vi "HFRR ADV v07 new software.vi"() -> ()   [LabVIEW 2025] (continued)
            n281 = call <vilib>:"Clear Errors.vi"("error in (no error)"=w363) -> ()  [unwired: 5 in, 2 out]
          }
          frame True {
          }
        }
      }
      event "Heater Button": Value Change {
        n282 = event-data() -> ()  [unwired: 1 in, 6 out]
        n283 = local read "Heater Button"() -> (w381:bool)
        n284 = case shown="True" w381 {
          frame True {
            n285 = stacked-sequence {
              frame #0 {
                n286 = Wait (ms)(milliseconds to wait=u32 1500) -> ()  [unwired: 1 out]
              }
              frame #1 {
                n287 = local read "Set Temp"() -> (w383:dbl)
                n288 = Number To Fractional String(number=w383, precision (6)=i16 2) -> (F-format string=w386:string)  [unwired: 2 in]
                n289 = Concatenate Strings("ST;" ("Command"), w386) -> (w385:string)
                n290 = local write "Command"(w385) -> ()
              }
              frame #2 {
                n291 = Wait (ms)(milliseconds to wait=u32 1500) -> ()  [unwired: 1 out]
              }
              frame #3 {
                n292 = local write "Command"("HE;1" ("Command")) -> ()
              }
              frame #4 {
                n293 = Wait (ms)(milliseconds to wait=u32 1500) -> ()  [unwired: 1 out]
              }
            }
          }
          frame False {
            n294 = stacked-sequence {
              frame #0 {
                n295 = Wait (ms)(milliseconds to wait=u32 1500) -> ()  [unwired: 1 out]
              }
              frame #1 {
                n296 = Concatenate Strings("ST;" ("Command"), "0" ("string")) -> (w393:string)
                n297 = local write "Command"(w393) -> ()
              }
              frame #2 {
                n298 = Wait (ms)(milliseconds to wait=u32 1500) -> ()  [unwired: 1 out]
              }
              frame #3 {
                n299 = local write "Command"("HE;0" ("Command")) -> ()
              }
              frame #4 {
                n300 = Wait (ms)(milliseconds to wait=u32 1500) -> ()  [unwired: 1 out]
              }
            }
          }
        }
      }
      event "Headen Service Button": Value Change {
        n301 = event-data() -> ()  [unwired: 1 in, 6 out]
        n302 = local read "Headen Service Button"() -> (w398:bool)
        n303 = case shown="True" w398 {
          frame False {
            n304 = property on="Password 3" class="Clust (strict)"("Visible"=FALSE) -> ()  [unwired: 2 in, 2 out]
            n305 = property on="Service Password Log" class="Str"("Visible"=FALSE) -> ()  [unwired: 2 in, 2 out]
          }
          frame True {
            n306 = property on="Password 3" class="Clust (strict)"("Visible"=TRUE) -> ()  [unwired: 2 in, 2 out]
            n307 = property on="Service Password Log" class="Str"("Visible"=TRUE) -> ()  [unwired: 2 in, 2 out]
          }
        }
      }
      event "Password 3.Service Password": Value Change {
        n308 = event-data() -> ()  [unwired: 1 in, 6 out]
        n309 = Unbundle By Name("Password 3") -> ("Service Password"=w405:string)
        n310 = call <vilib>:"Trim Whitespace.vi"("string"=w405) -> ("trimmed string"=w403:string)  [unwired: 1 in]
        n311 = Equal?(x=w403, y="Service@123") -> (x = y?=w404:bool)
        n312 = case shown="False" w404 {
          selector: w404 -> [w409 w411]
          frame False {
            n313 = local write "Service Password enable"(w409) -> ()
            n314 = property on="Service Password Log" class="Str"("Visible"=TRUE) -> ()  [unwired: 2 in, 2 out]
            n315 = property on="Tab Control 5" class="TabCtl (strict)"("Tabs Visible?"=TRUE ("Page Labels Display Visible?")) -> ()  [unwired: 2 in, 2 out]
          }
          frame True {
            n316 = property on="Service Password Log" class="Str"("Visible"=FALSE) -> ()  [unwired: 2 in, 2 out]
            "Service Password enable" <- w411
          }
        }
      }
      event "Sign In": Value Change {
        w413 = FALSE ("Visible")
        n317 = event-data() -> ()  [unwired: 1 in, 6 out]
        n318 = property on="About" class="Clust (strict)"("Visible"=w413) -> ()  [unwired: 2 in, 2 out]
        n319 = property on="Password 3" class="Clust (strict)"("Visible"=w413) -> ()  [unwired: 2 in, 2 out]
        n320 = property on="Service Password Log" class="Str"("Visible"=FALSE) -> ()  [unwired: 2 in, 2 out]
      }
      event "Info": Value Change {
        n321 = event-data() -> ()  [unwired: 1 in, 6 out]
        n322 = local read "Info"() -> (w415:bool)
        n323 = case shown="False" w415 {
          frame False {
            n324 = property on="About" class="Clust (strict)"("Visible"=FALSE) -> ()  [unwired: 2 in, 2 out]
          }
          frame True {
            n325 = property on="About" class="Clust (strict)"("Visible"=TRUE) -> ()  [unwired: 2 in, 2 out]
          }
        }
      }
      event "Calibration": Value Change {
        n326 = event-data() -> ()  [unwired: 1 in, 6 out]
        n327 = local read "Calibration"() -> (w419:bool)
        n328 = case shown="False" w419 {
          frame False {
            n329 = property on="Calibration 2" class="TabCtl (strict)"("Visible"=FALSE) -> ()  [unwired: 2 in, 2 out]
            n330 = local write "Cal Password"("" ("Cal Password")) -> ()
          }
          frame True {
            n331 = property on="Calibration 2" class="TabCtl (strict)"("Visible"=TRUE) -> ()  [unwired: 2 in, 2 out]
            n332 = local write "Cal Password"("" ("Cal Password")) -> ()
          }
        }
        n333 = property on="Wrong Password" class="Str"("Visible"=FALSE) -> ()  [unwired: 2 in, 2 out]
      }
      event "Cal Password": Value Change {
        n334 = event-data() -> ()  [unwired: 1 in, 6 out]
        n335 = local read "Cal Password"() -> (w427:string)
        n336 = call <vilib>:"Trim Whitespace.vi"("string"=w427) -> ("trimmed string"=w426:string)  [unwired: 1 in]
        n337 = Equal?(x=w426, y="Cal@321") -> (x = y?=w424:bool)
        n338 = case shown="True" w424 {
          frame False {
            n339 = property on="Wrong Password" class="Str"("Visible"=TRUE) -> ()  [unwired: 2 in, 2 out]
          }
          frame True {
            n340 = property on="Wrong Password" class="Str"("Visible"=FALSE) -> ()  [unwired: 2 in, 2 out]
            n341 = local write "Main Tab"(T2."About" ("Main Tab")) -> ()
            n342 = local write "Cal Password"("" ("Cal Password")) -> ()
            n343 = local write "Main Dashboard Buttons"(T1."About" ("Main Dashboard Buttons")) -> ()
            n344 = local write "Tab Control 5"(T9."Temperature Calibration" ("Tab Control 5")) -> ()
            n345 = property on="Calibration 2" class="TabCtl (strict)"("Visible"=FALSE) -> ()  [unwired: 2 in, 2 out]
            n346 = property on="Tab Control 5" class="TabCtl (strict)"("Tabs Visible?"=FALSE ("Page Labels Display Visible?")) -> ()  [unwired: 2 in, 2 out]
            n347 = local write "Calibration"(FALSE ("Calibration")) -> ()
          }
        }
      }
      event "Quit": Value Change {
        n348 = event-data() -> ()  [unwired: 1 in, 6 out]
      }
    }
    n349 = Wait (ms)(milliseconds to wait=u32 100) -> ()  [unwired: 1 out]
  }
  n350 = local write "Auto stop temp"(w14) -> ()
  n351 = local write "main tab sub"(enum32{"Page 1", "Page 2"}."Page 1" ("main tab sub")) -> ()
  n352 = local write "USERNAME"(w31) -> ()
  n353 = local write "Main Tab"(T2."HOME" ("Main Tab")) -> ()
  n354 = local write "USER ID"(w31) -> ()
  n355 = property on="Auto Scar Check  2" class="Clust (strict)"("Visible"=w14) -> (error out=w17:errorcluster)  [unwired: 2 in, 1 out]
  n356 = property on="Quit" class="Bool (strict)"("Value"=FALSE ("Quit")) -> (error out=w33:errorcluster)  [unwired: 2 in, 1 out]
  n357 = while {
    shift-right: [w439] -> _
    shift-left: "Enum - Selector" -> [w440]
    stop <- w441 stop-if-true
    # "Auto Start Logic Loop"
    n358 = case shown="\"close\"" w440 {
      tunnel: [w444 w450 w462 w494 w525 Auto_Start_enum."Exit" ("Enum - Selector") Auto_Start_enum."Init" ("Enum - Selector")] -> w439
      frame "Init", Default {
        n359 = local read "Auto Start Test"() -> (w443:bool)
        n360 = Select(t=Auto_Start_enum."Humidity & Temperature On" ("Enum - Selector"), s=w443, f=Auto_Start_enum."Init") -> (s? t:f=w444:T12)
      }
      frame "Humidity & Temperature On" {
        n361 = flat-sequence {
          tunnel: [Auto_Start_enum."Reach point" ("Enum - Selector")] -> w447
          frame #0 {
            w452 = T15."Disabled and Grayed Out" ("Disabled")
            w453 = TRUE ("Heater Button")
            n362 = property on="Humidity" class="Bool (strict)"("DisabledEnum"=w452) -> ()  [unwired: 2 in, 2 out]
            n363 = property on="Heater Button" class="Bool (strict)"("DisabledEnum"=w452) -> ()  [unwired: 2 in, 2 out]
            n364 = local write "Heater Button"(w453) -> ()
            n365 = local write "Humidity"(w453) -> ()
            n366 = property on="Heater Button" class="Bool (strict)"("Val(Sgnl)"=TRUE ("Value (Signaling)")) -> ()  [unwired: 2 in, 2 out]
          }
          frame #1 {
            n367 = Wait (ms)(milliseconds to wait=u32 3000) -> ()  [unwired: 1 out]
          }
          frame #2 {
            w455 = TRUE ("Reach point temp")
            n368 = local write "Reach point Humidity"(w455) -> ()
            n369 = local write "Reach point temp"(w455) -> ()
          }
        }
        n370 = local read "Auto Start Test"() -> (w449:bool)
        n371 = Not(x=w449) -> (.not. x?=w448:bool)
        n372 = Select(t=Auto_Start_enum."close", s=w448, f=w447) -> (s? t:f=w450:T12)
      }
      frame "Reach point" {
        w463 = TRUE ("PAUSE")
        w471 = 1.0 ("y")
        w474 = 1.0 ("y")
        n373 = local read "Set Temperature:"() -> (w475:dbl)
        n374 = local read "Set Humidity:"() -> (w470:dbl)
        n375 = local read "Humidity ( %RH )"() -> (w476:dbl)
        n376 = Add(x=w475, y=w474) -> (x+y=w473:dbl)
        n377 = Subtract(x=w475, y=w474) -> (x-y=w472:dbl)
        n378 = Add(x=w470, y=w471) -> (x+y=w469:dbl)
        n379 = Subtract(x=w470, y=w471) -> (x-y=w468:dbl)
        n380 = local read "TEMP"() -> (w477:dbl)
        n381 = In Range and Coerce(upper limit=w469, x=w476, lower limit=w468) -> (In Range?=w457:bool)  [unwired: 1 out]
        n382 = In Range and Coerce(upper limit=w473, x=w477, lower limit=w472) -> (In Range?=w458:bool)  [unwired: 1 out]
        n383 = case shown="True" w457 {
          frame False {
          }
          frame True {
            n384 = case shown="True" "Reach point Humidity" {
              selector: "Reach point Humidity" -> [_ w483]
              frame False {
              }
              frame True {
                n385 = local read "EVENT LOG"() -> (w480:string)
                n386 = Not(x=w483) -> (.not. x?=w482:bool)
                n387 = local write "Reach point Humidity"(w482) -> ()
                n388 = call "Event Log.vi"("Content"="Target Humidity reached", "EVENT LOG"=w480) -> ("EVENT LOG"=w481:string)  [unwired: 8 in, 1 out]
                n389 = local write "EVENT LOG"(w481) -> ()
              }
            }
          }
        }
        n390 = case shown="True" w458 {
          frame False {
          }
          frame True {
            n391 = case shown="True" "Reach point temp" {
              selector: "Reach point temp" -> [_ w489]
              frame False {
              }
              frame True {
                n392 = local read "EVENT LOG"() -> (w486:string)
                n393 = Not(x=w489) -> (.not. x?=w488:bool)
                n394 = local write "Reach point temp"(w488) -> ()
                n395 = call "Event Log.vi"("Content"="Target Temperature reached", "EVENT LOG"=w486) -> ("EVENT LOG"=w487:string)  [unwired: 8 in, 1 out]
                n396 = local write "EVENT LOG"(w487) -> ()
              }
            }
          }
        }
        n397 = local read "Auto Start Test"() -> (w461:bool)
        n398 = And(x=w458, y=w457) -> (x .and. y?=w467:bool)
        n399 = Select(t=Auto_Start_enum."Maintain Stage" ("Enum - Selector"), s=w467, f=Auto_Start_enum."Reach point" ("Enum - Selector")) -> (s? t:f=w464:T12)
        n400 = Not(x=w461) -> (.not. x?=w460:bool)
        n401 = Select(t=Auto_Start_enum."close", s=w460, f=w464) -> (s? t:f=w462:T12)
        n402 = call "ELAPSED TIMER VI.vi"("RESET"=w463, "PAUSE"=w463) -> ()  [unwired: 7 in, 3 out]
      }
      frame "Maintain Stage" {
        w503 = 2.0 ("y")
        w502 = 1.0 ("y")
        # "Humidity and  temperatures Set Point  have been reached"
        n403 = local read "Set Temperature:"() -> (w509:dbl)
        n404 = local read "Set Humidity:"() -> (w506:dbl)
        n405 = local read "Humidity ( %RH )"() -> (w510:dbl)
        n406 = Add(x=w509, y=w502) -> (x+y=w508:dbl)
        n407 = Subtract(x=w509, y=w502) -> (x-y=w507:dbl)
        n408 = local read "TEMP"() -> (w511:dbl)
        n409 = Add(x=w506, y=w503) -> (x+y=w505:dbl)
        n410 = Subtract(x=w506, y=w503) -> (x-y=w504:dbl)
        n411 = In Range and Coerce(upper limit=w508, x=w511, lower limit=w507) -> (In Range?=w501:bool)  [unwired: 1 out]
        n412 = In Range and Coerce(upper limit=w505, x=w510, lower limit=w504) -> (In Range?=w500:bool)  [unwired: 1 out]
        n413 = And(x=w501, y=w500) -> (x .and. y?=w499:bool)
        n414 = Not(x=w499) -> (.not. x?=w498:bool)
        n415 = call "ELAPSED TIMER VI.vi"("TARGET"=60.0, "RESET"=w498, "PAUSE"=FALSE) -> ("ELAPSED INDICATION"=w495:bool)  [unwired: 6 in, 2 out]
        n416 = case shown="True" w495 {
          tunnel: w495 -> [_ w514]
          tunnel: [Auto_Start_enum."Maintain Stage" ("Enum - Selector") w513] -> w493
          frame False {
          }
          frame True {
            n417 = stacked-sequence {
              tunnel: w514 -> [_ _ _ _ _]
              tunnel: [_ _ _ _ Auto_Start_enum."Start Stage" ("Enum - Selector")] -> w513
              frame #0 {
                n418 = local read "EVENT LOG"() -> (w516:string)
                n419 = call "Event Log.vi"("Content"="Humidity and temperature set point has stabilized.", "EVENT LOG"=w516) -> ("EVENT LOG"=w517:string)  [unwired: 8 in, 1 out]
                n420 = local write "EVENT LOG"(w517) -> ()
              }
              frame #1 {
                n421 = Wait (ms)(milliseconds to wait=u32 100) -> ()  [unwired: 1 out]
              }
              frame #2 {
                n422 = local read "EVENT LOG"() -> (w520:string)
                n423 = call "Event Log.vi"("Content"="Auto Test Started", "EVENT LOG"=w520) -> ("EVENT LOG"=w521:string)  [unwired: 8 in, 1 out]
                n424 = local write "EVENT LOG"(w521) -> ()
              }
              frame #3 {
                w522 = TRUE ("RUN")
                n425 = local write "RUN"(w522) -> ()
                "Auto Start Temp" <- w522
              }
              frame #4 {
              }
            }
          }
        }
        n426 = local read "Auto Start Test"() -> (w492:bool)
        n427 = Not(x=w492) -> (.not. x?=w491:bool)
        n428 = Select(t=Auto_Start_enum."close", s=w491, f=w493) -> (s? t:f=w494:T12)
      }
      frame "Start Stage" {
        w524 = TRUE ("PAUSE")
        n429 = local read "Auto Start Test"() -> (w529:bool)
        n430 = Not(x=w529) -> (.not. x?=w528:bool)
        n431 = Select(t=Auto_Start_enum."close" ("Enum - Selector"), s=w528, f=Auto_Start_enum."Start Stage" ("Enum - Selector")) -> (s? t:f=w525:T12)
        n432 = call "ELAPSED TIMER VI.vi"("RESET"=w524, "PAUSE"=w524) -> ()  [unwired: 7 in, 3 out]
      }
      frame "close" {
        w531 = FALSE ("Heater Button")
        n433 = local write "RUN"(w531) -> ()
        n434 = local write "Heater Button"(w531) -> ()
        n435 = local write "Humidity"(w531) -> ()
        n436 = local write "Auto Start Test"(w531) -> ()
        n437 = property on="Heater Button" class="Bool (strict)"("Val(Sgnl)"=FALSE ("Value (Signaling)")) -> ()  [unwired: 2 in, 2 out]
      }
      frame "Exit" {
      }
    }
    n438 = Wait (ms)(milliseconds to wait=u32 100) -> ()  [unwired: 1 out]
    n439 = local read "Quit"() -> (w441:bool)
  }
  n440 = property on="Service Password Log" class="Str"("Visible"=w14) -> ()  [unwired: 2 in, 2 out]
  n441 = property on="Password 3" class="Clust (strict)"("Visible"=w14) -> ()  [unwired: 2 in, 2 out]
  n442 = while {
    stop <- w560 stop-if-true
    w543 = errorcluster {"status"=FALSE, "code"=0, "source"=""} ("error in (no error) 3")
    # "this loop is for manual report generation"
    n443 = local read "Confirm Measrurement"() -> (w542:bool)
    n444 = case shown="True" w542 {
      selector: w542 -> [_ w650]
      tunnel: errorcluster {"status"=FALSE, "code"=0, "source"=""} ("error in (no error) 3") -> [_ w651]
      tunnel: [_ w649] -> _
      frame False {
      }
      frame True {
        n445 = stacked-sequence {
          tunnel: w651 -> [_ w684 _]
          tunnel: w650 -> [_ _ w791]
          tunnel: [_ w672 _] -> w649
          frame #0 {
            n446 = String To Path(string="C:\\LAB-IQ\\Image Calibrate v01.dcf") -> (path=w654:path)
            n447 = Open/Create/Replace File ("Open File")(file path (use dialog)=w654) -> (refnum out=w655:refnum<file>)  [unwired: 5 in, 2 out]
            n448 = for {
              N: 4 -> [_]
              tunnel: w655 -> [w661]
              i -> [w657]
              n449 = Read from Text File ("Read File")(file (use dialog)=w661) -> (text=w662:string)  [unwired: 3 in, 3 out]
              n450 = String Subset(string=w662, offset (0)=6, length (rest)=10 ("length (rest)")) -> (substring=w658:string)
              n451 = Fract/Exp String To Number(string=w658) -> (number=w656:dbl)  [unwired: 3 in, 1 out]
              n452 = case shown="3" w657 {
                tunnel: w656 -> [w663 w664 _ w665 _]
                frame 0 {
                  n453 = local write "5x Gain"(w663) -> ()
                }
                frame 1 {
                  n454 = local write "10x Gain"(w664) -> ()
                }
                frame 2 {
                }
                frame 3 {
                  n455 = local write "100x gain"(w665) -> ()
                }
                frame 4, Default {
                }
              }
            }
          }
          frame #1 {
            n456 = local read "TEST STANDARD"() -> (w667:T3)
            n457 = case shown="\"ISO 12156\"" w667 {
              tunnel: ["ASTM D6079" "ISO 12156"] -> w666
              frame "ASTM D6079", Default {
              }
              frame "ISO 12156" {
              }
            }
            n458 = call "IMAGE ANALYSIS.vi"("Enum"=POST_ANALYSIS_ENUM."GET MEASUREMENTS", "error in"=w684) -> ("error out"=w691:errorcluster)  [unwired: 8 in, 1 out]
            n459 = local read "Magnification :"() -> (w677:string)
            n460 = call "Stall Data Flow.vim"("value in"=w691, "milliseconds to wait"=u32 1000) -> ("value out"=w690:errorcluster)  [unwired: 1 out]
            n461 = local read "Test File List :"() -> (w688:string)
            n462 = case shown="\"10x\"" w677 {
              tunnel: [w727 w728] -> w675
              frame "5x", Default {
                n463 = local read "5x Gain"() -> (w727:dbl)
              }
              frame "10x" {
                # "5x"
                n464 = local read "10x Gain"() -> (w728:dbl)
              }
            }
            n465 = call "IMAGE ANALYSIS.vi"("Enum"=POST_ANALYSIS_ENUM."READ", "error in"=w690) -> ("error out"=w687:errorcluster, "data out"=w678:string)  [unwired: 8 in]
            n466 = Match Pattern(string=w678, regular expression="\"type\": ") -> (after substring=w682:string)  [unwired: 1 in, 3 out]
            n467 = call "IMAGE PATH CREATION PY.vi"("error in (no error)"=w687, "File Name :"=w688) -> ("error out"=w686:errorcluster, "File Path"=w674:path, "File Path String:"=w669:string)  [unwired: 7 in]
            n468 = Match Pattern(string=w682, regular expression=",") -> (before substring=w668:string)  [unwired: 1 in, 3 out]
            n469 = local read "Calibration Tab"() -> (w671:enum32{"Measrument", "Calibrate"})
            n470 = call "Stall Data Flow.vim"("value in"=w686, "milliseconds to wait"=u32 250) -> ("value out"=w670:errorcluster)  [unwired: 1 out]
            n471 = Equal?(x=w668, y="\"rectangle\"") -> (x = y?=w679:bool)
            n472 = case shown="False" w679 {
              tunnel: w678 -> [w733 w788]
              tunnel: w675 -> [_ w779]
              tunnel: cluster{"major":dbl, "minor":dbl, "average":dbl} {"major"=0.0, "minor"=0.0, "average"=0.0} -> [w731 w775]
              tunnel: [w730 w772] -> w673
              tunnel: w668 -> [w732 _]
              tunnel: w675 -> [w729 _]
              frame False {
                n473 = Equal?(x=w732, y="\"line\"") -> (x = y?=w734:bool)
                n474 = case shown="True" w734 {
                  tunnel: w733 -> [_ w749]
                  tunnel: w731 -> [w736 w748]
                  tunnel: [w736 w746] -> w730
                  tunnel: w729 -> [_ w745]
                  frame False {
                  }
                  frame True {
                    w744 = 0.0 ("Major Axis")
                    n475 = Match Pattern(string=w749, regular expression="\"length_px\":") -> (after substring=w747:string)  [unwired: 1 in, 3 out]
                    n476 = property on="Major Axis" class="DigNum (strict)"("Caption.Text"="") -> ()  [unwired: 2 in, 2 out]
                    n477 = property on="Minor Axis" class="DigNum (strict)"("Caption.Text"="") -> ()  [unwired: 2 in, 2 out]
                    n478 = property on="Average" class="DigNum (strict)"("Caption.Text"="Line") -> ()  [unwired: 2 in, 2 out]
                    n479 = Fract/Exp String To Number(string=w747, default (0 dbl)=0.0 ("default (0 DBL)")) -> (number=w743:dbl)  [unwired: 2 in, 1 out]
                    "Pixel Value" <- w743
                    n480 = Multiply(x=w743, y=w745) -> (x*y=w756:dbl)
                    n481 = Multiply(x=w756, y=1000.0) -> (x*y=w739:dbl)
                    n482 = Divide(x=w739, y=1000.0) -> (x/y=w742:dbl)
                    n483 = local write "Measurment (mm)"(w742) -> ()
                    n484 = Bundle By Name(cluster=w748, "average"=w739) -> (w746:cluster{"major":dbl, "minor":dbl, "average":dbl})
                    n485 = Number To Fractional String(number=w739, precision (6)=i16 1) -> (F-format string=w738:string)  [unwired: 2 in]
                    n486 = local write "Minor Axis"(w744) -> ()
                    n487 = local write "Major Axis"(w744) -> ()
                    n488 = Fract/Exp String To Number(string=w738) -> (number=w737:dbl)  [unwired: 3 in, 1 out]
                    n489 = local write "Average"(w737) -> ()
                  }
                }
              }
              frame True {
                w776 = 1000.0 ("y")
                w782 = 0.0 ("default (0 DBL)")
                n490 = Match Pattern(string=w788, regular expression=" \"width_px\":") -> (after substring=w786:string)  [unwired: 1 in, 3 out]
                n491 = Match Pattern(string=w786, regular expression="\"height_px\":") -> (before substring=w784:string, after substring=w783:string)  [unwired: 1 in, 2 out]
                n492 = Fract/Exp String To Number(string=w784, default (0 dbl)=w782) -> (number=w781:dbl)  [unwired: 2 in, 1 out]
                n493 = Fract/Exp String To Number(string=w783, default (0 dbl)=w782) -> (number=w780:dbl)  [unwired: 2 in, 1 out]
                n494 = Multiply(x=w781, y=w779) -> (x*y=w778:dbl)
                n495 = Multiply(x=w780, y=w779) -> (x*y=w777:dbl)
                n496 = Multiply(x=w778, y=w776) -> (x*y=w762:dbl)
                n497 = Multiply(x=w777, y=w776) -> (x*y=w760:dbl)
                n498 = Add(x=w762, y=w760) -> (x+y=w774:dbl)
                n499 = property on="Major Axis" class="DigNum (strict)"("Caption.Text"="Major Axis") -> ()  [unwired: 2 in, 2 out]
                n500 = property on="Minor Axis" class="DigNum (strict)"("Caption.Text"="Minor Axis") -> ()  [unwired: 2 in, 2 out]
                n501 = property on="Average" class="DigNum (strict)"("Caption.Text"="Average") -> ()  [unwired: 2 in, 2 out]
                n502 = Divide(x=w774, y=2.0) -> (x/y=w758:dbl)
                n503 = Bundle By Name(cluster=w775, "major"=w762, "minor"=w760, "average"=w758) -> (w772:cluster{"major":dbl, "minor":dbl, "average":dbl})
                n504 = Number To Fractional String(number=w760, precision (6)=i16 1) -> (F-format string=w767:string)  [unwired: 2 in]
                n505 = Number To Fractional String(number=w758, precision (6)=i16 1) -> (F-format string=w768:string)  [unwired: 2 in]
                n506 = Number To Fractional String(number=w762, precision (6)=i16 1) -> (F-format string=w766:string)  [unwired: 2 in]
                n507 = Fract/Exp String To Number(string=w767) -> (number=w759:dbl)  [unwired: 3 in, 1 out]
                n508 = Fract/Exp String To Number(string=w768) -> (number=w757:dbl)  [unwired: 3 in, 1 out]
                n509 = Fract/Exp String To Number(string=w766) -> (number=w761:dbl)  [unwired: 3 in, 1 out]
                n510 = local write "Major Axis"(w761) -> ()
                n511 = local write "Average"(w757) -> ()
                n512 = local write "Minor Axis"(w759) -> ()
              }
            }
            n513 = case shown="\"Measrument\", Default" w671 {
              tunnel: w674 -> [w701 _]
              tunnel: w673 -> [w700 _]
              tunnel: [w697 w726] -> w672
              tunnel: w670 -> [w699 w726]
              tunnel: w669 -> [w698 _]
              tunnel: w666 -> [w696 _]
              frame "Measrument", Default {
                n514 = stacked-sequence {
                  tunnel: w701 -> [w719 _]
                  tunnel: w700 -> [w717 _]
                  tunnel: w699 -> [w715 _]
                  tunnel: w698 -> [w714 _]
                  tunnel: [w709 _] -> w697
                  tunnel: w696 -> [w702 _]
                  frame #0 {
                    n515 = call "IMAGE ANALYSIS.vi"("Enum"=POST_ANALYSIS_ENUM."SAVE IMAGE", "error in"=w715, "IMAGE FILE PATH"=w714) -> ("error out"=w713:errorcluster)  [unwired: 7 in, 1 out]
                    n516 = call "Stall Data Flow.vim"("value in"=w713, "milliseconds to wait"=u32 1000) -> ("value out"=w704:errorcluster)  [unwired: 1 out]
                    n517 = local read "Test File List :"() -> (w721:string)
                    n518 = call "IMAGE ANALYSIS.vi"("Enum"=POST_ANALYSIS_ENUM."MINIMIZE UI", "error in"=w704) -> ("error out"=w711:errorcluster)  [unwired: 8 in, 1 out]
                    n519 = Bundle By Name(cluster=T22 {"File Name"="", "Test Method"="", "Operator"="", "Fuel Description"="", "Date and time"=""} ("Main Ref"), "Test Method"=w702, "File Name"=w721) -> (w722:T22)
                    n520 = call "Stall Data Flow.vim"("value in"=w711, "milliseconds to wait"=u32 1500) -> ("value out"=w706:errorcluster)  [unwired: 1 out]
                    n521 = call "duf file read.vi"("error in (no error)"=w706, "Main Ref"=w722) -> ("error out"=w720:errorcluster, "Main Ref 2"=w718:T22)  [unwired: 8 in]
                    n522 = call "DETECTION REPORT for manual.vi"("error in (no error)"=w720, "return value 3"=w717, "Image File Path"=w719, "Main Ref"=w718) -> ("error out"=w716:errorcluster)  [unwired: 7 in]
                    n523 = call <vilib>:"Clear Errors.vi"("error in (no error)"=w716) -> ("error out"=w707:errorcluster)  [unwired: 5 in, 1 out]
                    n524 = call "IMAGE ANALYSIS.vi"("Enum"=POST_ANALYSIS_ENUM."MINIMIZE UI", "error in"=w707) -> ("error out"=w709:errorcluster)  [unwired: 8 in, 1 out]
                  }
                  frame #1 {
                    n525 = local write "Main Tab"(T2."HOME" ("Main Tab")) -> ()
                    n526 = local write "Main Dashboard Buttons"(T1."Home" ("Main Dashboard Buttons")) -> ()
                  }
                }
              }
              frame "Calibrate" {
              }
            }
          }
          frame #2 {
            n527 = Not(x=w791) -> (.not. x?=w790:bool)
            n528 = local write "Confirm Measrurement"(w790) -> ()
            n529 = local read "Calibration Tab"() -> (w789:enum32{"Measrument", "Calibrate"})
            n530 = case shown="\"Measrument\", Default" w789 {
              frame "Measrument", Default {
                (unwired) T17."HOME" ("Main Tab")
                n531 = local write "Main Tab"(T2."HOME" ("Main Tab")) -> ()
              }
              frame "Calibrate" {
              }
            }
          }
        }
      }
    }
    n532 = local read "Humidity"() -> (w534:bool)
    n533 = local read "Save Change"() -> (w539:bool)
    n534 = local read "Calibrate"() -> (w540:bool)
    n535 = local read "Auto Start Test"() -> (w535:bool)
    n536 = case shown="True" w540 {
      selector: w540 -> [_ w647]
      frame False {
      }
      frame True {
        n537 = Not(x=w647) -> (.not. x?=w646:bool)
        n538 = local write "Calibrate"(w646) -> ()
        n539 = local write "Calibration Tab"(enum32{"Measrument", "Calibrate"}."Calibrate" ("Calibration Tab")) -> ()
      }
    }
    n540 = case shown="True" w539 {
      selector: w539 -> [_ w591]
      frame False {
      }
      frame True {
        n541 = stacked-sequence {
          tunnel: w591 -> [_ _ _ _ w645]
          frame #0 {
            n542 = call "IMAGE ANALYSIS.vi"("Enum"=POST_ANALYSIS_ENUM."HIDE UI") -> ()  [unwired: 9 in, 2 out]
          }
          frame #1 {
            n543 = local read "100x gain"() -> (w593:dbl)
            n544 = local read "10x Gain"() -> (w594:dbl)
            n545 = local read "5x Gain"() -> (w595:dbl)
            n546 = Number To Fractional String(number=w594, width (-)=i16 4, precision (6)=i16 7) -> (F-format string=w616:string)  [unwired: 1 in]
            n547 = Number To Fractional String(number=0.0, width (-)=i16 4, precision (6)=i16 7) -> (F-format string=w611:string)  [unwired: 1 in]
            n548 = Number To Fractional String(number=w593, width (-)=i16 4, precision (6)=i16 7) -> (F-format string=w599:string)  [unwired: 1 in]
            n549 = Number To Fractional String(number=w595, width (-)=i16 10 ("precision (6)"), precision (6)=i16 7) -> (F-format string=w625:string)  [unwired: 1 in]
            n550 = Concatenate Strings("[CH1]" ("string"), w625, " - 5x Gain" ("string"), "\r") -> (w615:string)
            n551 = Concatenate Strings("[CH2]" ("string"), w616, " - 10x Gain" ("string"), "\r") -> (w614:string)
            n552 = Concatenate Strings("[CH3]" ("string"), w611, " - 20x Gain" ("string"), "\r") -> (w605:string)
            n553 = Concatenate Strings("[CH4]" ("string"), w599, " - 100x Gain" ("string"), "\r") -> (w598:string)
            n554 = String To Path(string="C:\\LAB-IQ\\Image Calibrate v01.dcf") -> (path=w628:path)
            n555 = Concatenate Strings(w615, w614, w605, w598) -> (w613:string)
            n556 = call <vilib>:"Write Characters To File.vi"("append to file? (new file:F)"=FALSE, "character string"=w613, "file path (dialog if empty)"=w628) -> ()  [unwired: 2 in, 1 out]
          }
          frame #2 {
            n557 = String To Path(string="C:\\LAB-IQ\\Image Calibrate v01.dcf") -> (path=w631:path)
            n558 = Open/Create/Replace File ("Open File")(file path (use dialog)=w631) -> (refnum out=w632:refnum<file>)  [unwired: 5 in, 2 out]
            n559 = for {
              N: 4 -> [_]
              tunnel: w632 -> [w638]
              i -> [w634]
              n560 = Read from Text File ("Read File")(file (use dialog)=w638) -> (text=w639:string)  [unwired: 3 in, 3 out]
              n561 = String Subset(string=w639, offset (0)=6, length (rest)=10 ("length (rest)")) -> (substring=w635:string)
              n562 = Fract/Exp String To Number(string=w635) -> (number=w633:dbl)  [unwired: 3 in, 1 out]
              n563 = case shown="3" w634 {
                tunnel: w633 -> [w640 w641 _ w642 _]
                frame 0 {
                  n564 = local write "5x Gain"(w640) -> ()
                }
                frame 1 {
                  n565 = local write "10x Gain"(w641) -> ()
                }
                frame 2 {
                }
                frame 3 {
                  n566 = local write "100x gain"(w642) -> ()
                }
                frame 4, Default {
                }
              }
            }
          }
          frame #3 {
            n567 = call "IMAGE ANALYSIS.vi"("Enum"=POST_ANALYSIS_ENUM."SHOW UI") -> ()  [unwired: 9 in, 2 out]
          }
          frame #4 {
            n568 = Not(x=w645) -> (.not. x?=w644:bool)
            n569 = local write "Save Change"(w644) -> ()
          }
        }
      }
    }
    n570 = case shown="False" w535 {
      tunnel: w534 -> [w561 _]
      frame False {
        n571 = case shown="True" w561 {
          frame False {
          }
          frame True {
            n572 = local read "Set Humidity:"() -> (w565:dbl)
            n573 = local read "Set Humidity:"() -> (w568:dbl)
            n574 = local read "Humidity ( %RH )"() -> (w569:dbl)
            n575 = Subtract(x=w565, y=2.0) -> (x-y=w563:dbl)
            n576 = Add(x=w568, y=2.0) -> (x+y=w564:dbl)
            n577 = In Range and Coerce(upper limit=w564, x=w569, lower limit=w563) -> (In Range?=w562:bool)  [unwired: 1 out]
            n578 = case shown="True" w562 {
              frame False {
              }
              frame True {
                n579 = case shown="False" "Manual Humididty Reached" {
                  selector: "Manual Humididty Reached" -> [_ w572]
                  frame False {
                  }
                  frame True {
                    n580 = Not(x=w572) -> (.not. x?=w571:bool)
                    n581 = local write "Manual Humididty Reached"(w571) -> ()
                    n582 = local read "EVENT LOG"() -> (w574:string)
                    n583 = call "Event Log.vi"("Content"="Target Humidity reached", "EVENT LOG"=w574) -> ("EVENT LOG"=w573:string)  [unwired: 8 in, 1 out]
                    n584 = local write "EVENT LOG"(w573) -> ()
                  }
                }
              }
            }
          }
        }
      }
      frame True {
        n585 = local write "Manual Humididty Reached"(TRUE ("Manual Humididty Reached")) -> ()
      }
    }
    n586 = local read "Cap Live Image"() -> (w555:bool)
    n587 = local read "SCAR MEASURMENT"() -> (w558:enum32{"Auto Scar", "Manual Scar"})
    n588 = Wait (ms)(milliseconds to wait=u32 250) -> ()  [unwired: 1 out]
    n589 = Equal?(x=w558, y=enum32{"Auto Scar", "Manual Scar"}."Manual Scar" ("SCAR MEASURMENT")) -> (x = y?=w556:bool)
    n590 = And(x=w556, y=w555) -> (x .and. y?=w554:bool)
    n591 = case shown="True" w554 {
      selector: w554 -> [_ w870]
      frame False {
      }
      frame True {
        n592 = stacked-sequence {
          tunnel: [_ _ _ w885 _] -> _
          tunnel: w870 -> [_ _ _ _ w892]
          frame #0 {
            w871 = 0.0
            n593 = local write "Major Axis"(w871) -> ()
            n594 = local write "Minor Axis"(w871) -> ()
            n595 = local write "Average"(w871) -> ()
          }
          frame #1 {
            n596 = call "CAMERA LIVE FEED FGV.vi"("Enum - Menu"=CAMERA_LIVE_FEED_ENUM."CAMERA MINIMIZE") -> ()  [unwired: 9 in, 2 out]
          }
          frame #2 {
            n597 = local read "FILE 3"() -> (w879:string)
            n598 = call <vilib>:"Trim Whitespace.vi"("string"="C:\\LAB-IQ\\images\\") -> ("trimmed string"=w881:string)  [unwired: 1 in]
            n599 = String To Path(string=w881) -> (path=w880:path)
            n600 = Concatenate Strings(w879, ".png" ("string")) -> (w878:string)
            n601 = Build Path(base path=w880, name or relative path=w878) -> (appended path=w876:path)
            n602 = Path To String(path=w876) -> (string=w875:string)
            n603 = call "CAMERA LIVE FEED FGV.vi"("Enum - Menu"=CAMERA_LIVE_FEED_ENUM."CAMERA SAVE", "Image Path"=w875) -> ("error out"=w873:errorcluster)  [unwired: 8 in, 1 out]
            n604 = case shown="No Error" w873 {
              frame No Error {
                n605 = One Button Dialog(message="Image saved successfully") -> ()  [unwired: 1 in, 1 out]
              }
              frame Error {
              }
            }
          }
          frame #3 {
            n606 = call "LIST FILE NAMES.vi"() -> ("error out"=w887:errorcluster, "filenames"=w884:string[])  [unwired: 10 in]
            n607 = call "IMAGE ANALYSIS.vi"("Enum"=POST_ANALYSIS_ENUM."SHOW UI", "error in"=w887) -> ("error out"=w885:errorcluster)  [unwired: 8 in, 1 out]
            n608 = property on="Test File List :" class="CmbBox"("Strings[]"=w884) -> ()  [unwired: 2 in, 2 out]
          }
          frame #4 {
            (unwired) T21."Report" ("Main Dashboard Buttons")
            (unwired) T23."Report" ("Main Dashboard Buttons")
            n609 = Not(x=w892) -> (.not. x?=w891:bool)
            n610 = local write "Zoom Factore"(0.0 ("Zoom Factore")) -> ()
            n611 = local write "Cap Live Image"(w891) -> ()
            n612 = local write "Main Tab"(T2."Adv Scar Report" ("Main Tab")) -> ()
            n613 = property on="Cap Live Image" class="Bool (strict)"("BoolText.Text"="Capture Image" ("Boolean Text.Text")) -> ()  [unwired: 2 in, 2 out]
            n614 = local write "Main Dashboard Buttons"(T1."Report" ("Main Dashboard Buttons")) -> ()
          }
        }
      }
    }
    n615 = local read "change Gain"() -> (w538:bool)
    n616 = local read "Back Square"() -> (w537:bool)
    n617 = case shown="True" w538 {
      selector: w538 -> [_ w582]
      frame False {
      }
      frame True {
        n618 = stacked-sequence {
          tunnel: w582 -> [_ w590]
          frame #0 {
            n619 = local read "Actual (µm)"() -> (w586:dbl)
            n620 = local read "Pixel Value"() -> (w585:dbl)
            n621 = local read "Magnification :"() -> (w584:string)
            n622 = Divide(x=w586, y=w585) -> (x/y=w583:dbl)
            n623 = case shown="\"10x\"" w584 {
              tunnel: w583 -> [w587 w588]
              frame "10x" {
                n624 = local write "10x Gain"(w587) -> ()
              }
              frame "5x", Default {
                n625 = local write "5x Gain"(w588) -> ()
              }
            }
          }
          frame #1 {
            n626 = Not(x=w590) -> (.not. x?=w589:bool)
            n627 = local write "change Gain"(w589) -> ()
          }
        }
      }
    }
    n628 = case shown="True" w537 {
      selector: w537 -> [_ w580]
      frame False {
      }
      frame True {
        n629 = Not(x=w580) -> (.not. x?=w579:bool)
        n630 = local write "Back Square"(w579) -> ()
        n631 = local write "Calibration Tab"(enum32{"Measrument", "Calibrate"}."Measrument" ("Calibration Tab")) -> ()
      }
    }
    n632 = local read "Rectangle Tool"() -> (w549:bool)
    n633 = local read "Clear ROI Tool"() -> (w548:bool)
    n634 = local read "Open Image"() -> (w553:bool)
    n635 = local read "line tool"() -> (w550:bool)
    n636 = local read "OUT"() -> (w551:bool)
    n637 = local read "In"() -> (w552:bool)
    n638 = case shown="True" w553 {
      selector: w553 -> [_ w858]
      tunnel: [w854 w860] -> _
      tunnel: w543 -> [w854 w859]
      frame False {
      }
      frame True {
        n639 = Not(x=w858) -> (.not. x?=w857:bool)
        n640 = local write "Open Image"(w857) -> ()
        n641 = call "IMAGE ANALYSIS.vi"("Enum"=POST_ANALYSIS_ENUM."HIDE UI", "error in"=w859) -> ("error out"=w867:errorcluster)  [unwired: 8 in, 1 out]
        n642 = call "File Dialog"("start path"=path "C:/LAB-IQ/images", "error in"=w867) -> ("selected path"=w856:path, "error out"=w865:errorcluster)  [unwired: 10 in, 2 out]
        "Image path  2" <- w856
        n643 = call <vilib>:"Clear Errors.vi"("error in (no error)"=w865) -> ("error out"=w864:errorcluster)  [unwired: 5 in, 1 out]
        n644 = call "IMAGE ANALYSIS.vi"("Enum"=POST_ANALYSIS_ENUM."OPEN FILE", "error in"=w864, "File Path"=w856) -> ("error out"=w863:errorcluster)  [unwired: 7 in, 1 out]
        n645 = call <vilib>:"Clear Errors.vi"("error in (no error)"=w863) -> ("error out"=w862:errorcluster)  [unwired: 5 in, 1 out]
        n646 = call "IMAGE ANALYSIS.vi"("Enum"=POST_ANALYSIS_ENUM."SHOW UI", "error in"=w862) -> ("error out"=w860:errorcluster)  [unwired: 8 in, 1 out]
        n647 = local write "Zoom Factore"(100.0 ("Zoom Factore")) -> ()
      }
    }
    n648 = case shown="True" w551 {
      selector: w551 -> [_ w839]
      tunnel: w543 -> [w836 w844]
      tunnel: [w836 w838] -> _
      frame False {
      }
      frame True {
        n649 = Not(x=w839) -> (.not. x?=w837:bool)
        n650 = local read "Zoom Factore"() -> (w842:dbl)
        n651 = local write "OUT"(w837) -> ()
        n652 = call "IMAGE ANALYSIS.vi"("Enum"=POST_ANALYSIS_ENUM."ZOOM OUT", "error in"=w844) -> ("error out"=w838:errorcluster)  [unwired: 8 in, 1 out]
        n653 = Divide(x=w842, y=1.2) -> (x/y=w840:dbl)
        n654 = local write "Zoom Factore"(w840) -> ()
      }
    }
    n655 = case shown="True" w552 {
      selector: w552 -> [_ w848]
      tunnel: w543 -> [w845 w853]
      tunnel: [w845 w846] -> _
      frame False {
      }
      frame True {
        n656 = Not(x=w848) -> (.not. x?=w847:bool)
        n657 = local read "Zoom Factore"() -> (w851:dbl)
        n658 = local write "In"(w847) -> ()
        n659 = call "IMAGE ANALYSIS.vi"("Enum"=POST_ANALYSIS_ENUM."ZOOM IN", "error in"=w853) -> ("error out"=w846:errorcluster)  [unwired: 8 in, 1 out]
        n660 = Multiply(x=w851, y=1.2) -> (x*y=w849:dbl)
        n661 = local write "Zoom Factore"(w849) -> ()
      }
    }
    n662 = case shown="True" w548 {
      selector: w548 -> [_ w820]
      tunnel: w543 -> [w818 w822]
      tunnel: [w818 w821] -> _
      frame False {
      }
      frame True {
        n663 = Not(x=w820) -> (.not. x?=w819:bool)
        n664 = local write "Clear ROI Tool"(w819) -> ()
        n665 = call "IMAGE ANALYSIS.vi"("Enum"=POST_ANALYSIS_ENUM."CLEAR ROI", "error in"=w822) -> ("error out"=w821:errorcluster)  [unwired: 8 in, 1 out]
      }
    }
    n666 = case shown="True" w550 {
      selector: w550 -> [_ w832]
      tunnel: w543 -> [w830 w835]
      tunnel: [w830 w833] -> _
      frame False {
      }
      frame True {
        n667 = Not(x=w832) -> (.not. x?=w831:bool)
        n668 = local write "line tool"(w831) -> ()
        n669 = call "IMAGE ANALYSIS.vi"("Enum"=POST_ANALYSIS_ENUM."DRAW LINE", "error in"=w835) -> ("error out"=w833:errorcluster)  [unwired: 8 in, 1 out]
      }
    }
    n670 = case shown="True" w549 {
      selector: w549 -> [_ w826]
      tunnel: w543 -> [w824 w828]
      tunnel: [w824 w827] -> _
      frame False {
      }
      frame True {
        n671 = Not(x=w826) -> (.not. x?=w825:bool)
        n672 = local write "Rectangle Tool"(w825) -> ()
        n673 = call "IMAGE ANALYSIS.vi"("Enum"=POST_ANALYSIS_ENUM."DRAW REC", "error in"=w828) -> ("error out"=w827:errorcluster)  [unwired: 8 in, 1 out]
      }
    }
    n674 = local read "SCAR MEASURMENT"() -> (w536:enum32{"Auto Scar", "Manual Scar"})
    n675 = local read "Fit to Screen Tool"() -> (w545:bool)
    n676 = local read "Resize Tool"() -> (w544:bool)
    n677 = case shown="\"Manual Scar\", Default" w536 {
      frame "Auto Scar" {
        n678 = property on="Cap Live Image" class="Bool (strict)"("BoolText.Text"="Report" ("Boolean Text.Text")) -> ()  [unwired: 2 in, 2 out]
      }
      frame "Manual Scar", Default {
        n679 = property on="Cap Live Image" class="Bool (strict)"("BoolText.Text"="Save Image" ("Boolean Text.Text")) -> ()  [unwired: 2 in, 2 out]
      }
    }
    n680 = local read "ROI Color Tool"() -> (w546:bool)
    n681 = local read "Pan Tool"() -> (w547:bool)
    n682 = case shown="True" w547 {
      selector: w547 -> [_ w814]
      tunnel: w543 -> [w812 w816]
      tunnel: [w812 w815] -> _
      frame False {
      }
      frame True {
        n683 = Not(x=w814) -> (.not. x?=w813:bool)
        n684 = call "IMAGE ANALYSIS.vi"("Enum"=POST_ANALYSIS_ENUM."PAN", "error in"=w816) -> ("error out"=w815:errorcluster)  [unwired: 8 in, 1 out]
        n685 = local write "Pan Tool"(w813) -> ()
      }
    }
    n686 = case shown="True" w544 {
      selector: w544 -> [_ w798]
      tunnel: w543 -> [w793 w795]
      tunnel: [w793 w794] -> _
      frame False {
      }
      frame True {
        n687 = Not(x=w798) -> (.not. x?=w797:bool)
        n688 = local write "Resize Tool"(w797) -> ()
        n689 = call "IMAGE ANALYSIS.vi"("Enum"=POST_ANALYSIS_ENUM."RESIZE MODE", "error in"=w795) -> ("error out"=w794:errorcluster)  [unwired: 8 in, 1 out]
      }
    }
    n690 = case shown="True" w545 {
      selector: w545 -> [_ w803]
      tunnel: [w799 w804] -> _
      tunnel: w543 -> [w799 w802]
      frame False {
      }
      frame True {
        n691 = Not(x=w803) -> (.not. x?=w801:bool)
        n692 = local write "Zoom Factore"(100.0 ("Zoom Factore")) -> ()
        n693 = local write "Fit to Screen Tool"(w801) -> ()
        n694 = call "IMAGE ANALYSIS.vi"("Enum"=POST_ANALYSIS_ENUM."FIT", "error in"=w802) -> ("error out"=w804:errorcluster)  [unwired: 8 in, 1 out]
      }
    }
    n695 = case shown="True" w546 {
      selector: w546 -> [_ w809]
      tunnel: [w806 w810] -> _
      tunnel: w543 -> [w806 w807]
      frame False {
      }
      frame True {
        n696 = Not(x=w809) -> (.not. x?=w808:bool)
        n697 = local write "ROI Color Tool"(w808) -> ()
        n698 = call "IMAGE ANALYSIS.vi"("Enum"=POST_ANALYSIS_ENUM."SET ROI COLOR", "error in"=w807) -> ("error out"=w810:errorcluster)  [unwired: 8 in, 1 out]
      }
    }
    n699 = local read "Quit"() -> (w560:bool)
  }
  n700 = while {
    stop <- w894 stop-if-true
    n701 = local read "Image Path"() -> (w897:path)
    n702 = local read "Print 3"() -> (w900:bool)
    n703 = Equal?(x=w897, y=path "") -> (x = y?=w896:bool)
    n704 = Not(x=w896) -> (.not. x?=w895:bool)
    n705 = property on="Print 3" class="Bool (strict)"("Visible"=w895) -> ()  [unwired: 2 in, 2 out]
    n706 = case shown="True" w900 {
      frame False {
        n707 = local write "Rd"(TRUE ("Boolean 7")) -> ()
      }
      frame True {
        n708 = flat-sequence {
          tunnel: [w940] -> w908
          tunnel: [w927] -> w906
          tunnel: [w937] -> w902
          tunnel: w908 -> [w949]
          tunnel: [w949] -> w907
          tunnel: w906 -> [w948]
          tunnel: [w948] -> w905
          tunnel: [w946] -> w904
          tunnel: [w945] -> w903
          tunnel: w902 -> [w945]
          tunnel: w907 -> [w951]
          tunnel: w905 -> [w952]
          tunnel: w904 -> [_]
          tunnel: w903 -> [w950]
          frame #0 {
            n709 = case shown="True" "Rd" {
              frame False {
              }
              frame True {
                n710 = while {
                  tunnel: "abcdefABCDEF" ("string 2") -> [w919]
                  shift-right: [w917] -> w911
                  shift-left: "" -> [w916]
                  i -> [w926]
                  stop <- w925 stop-if-true
                  n711 = Random Number (0-1)() -> (number: 0 to 1=w920:dbl)
                  n712 = Multiply(x=w920, y=62.0) -> (x*y=w922:dbl)
                  n713 = Decrement(x="Length 2") -> (x-1=w915:i16)
                  n714 = To Word Integer(number=w922) -> (16bit integer=w923:i16)
                  n715 = String Subset(string=w919, offset (0)=w923, length (rest)=1 ("length (rest)")) -> (substring=w918:string)
                  n716 = Greater Or Equal?(x=w926, y=w915) -> (x >= y?=w925:bool)
                  n717 = Concatenate Strings(w918, w916) -> (w917:string)
                }
                "String 10" <- w911
                n718 = local write "Rd"(FALSE ("Boolean 7")) -> ()
              }
            }
          }
          frame #1 {
            w938 = "_resized.jpg" ("command line")
            (unwired) ".jpg -resize 320x240 " ("string")
            (unwired) "Choose an Image File" ("prompt")
            # "-resize 1798x425"
            n719 = local read "Image Path"() -> (w932:path)
            n720 = Strip Path(path=w932) -> (stripped path=w927:path, name=w928:string)
            n721 = Match Pattern(string=w928, regular expression=".jpg") -> (before substring=→"before substring 2":string, after substring=→"after substring":string)  [unwired: 1 in, 2 out]
            n722 = Match Pattern(string=w928, regular expression="\\") -> (before substring=w934:string)  [unwired: 1 in, 3 out]
            n723 = Match Pattern(string=w934, regular expression=".jpg") -> (before substring=w933:string)  [unwired: 1 in, 3 out]
            n724 = Concatenate Strings("cmd /c convert " ("string"), w933, ".jpg -resize 320x240  " ("command line"), w933, w938) -> (w941:string)
            n725 = call <vilib>:"System Exec.vi"("run minimized? (F)"=TRUE, "wait until completion? (T)"=TRUE, "working directory"=w927, "command line"=w941) -> ("error out"=w940:errorcluster)  [unwired: 4 in, 3 out]
            "error out 2" <- w940
            n726 = Concatenate Strings(w933, w938) -> (w937:string)
          }
          frame #2 {
            n727 = Wait (ms)(milliseconds to wait=u32 2000 ("millisecond timer value")) -> (millisecond timer value=w946:u32)
          }
          frame #3 {
            n728 = case shown="No Error" w951 {
              tunnel: w952 -> [w955 _]
              tunnel: w950 -> [w953 _]
              frame No Error {
                (unwired) ".jpg" ("string")
                n729 = Path To String(path=w955) -> (string=w959:string)
                n730 = Concatenate Strings(w959, "\\" ("string"), w953) -> (w958:string)
                n731 = String To Path(string=w958) -> (path=w957:path)
                n732 = call <vilib>:"Read JPEG File.vi"("path to JPEG file"=w957) -> ("image data"=w961:T13)  [unwired: 8 in, 2 out]
                "image data" <- w961
                n733 = local write "Print 3"(FALSE ("Print 2")) -> ()
                n734 = call <vilib>:"Draw Flattened Pixmap.vi"("image data"=w961) -> ("new picture"=→"new picture":picture)  [unwired: 8 in]
              }
              frame Error {
              }
            }
          }
        }
      }
    }
    n735 = Wait (ms)(milliseconds to wait=u32 20 ("millisecond timer value")) -> ()  [unwired: 1 out]
    n736 = local read "Quit"() -> (w894:bool)
  }
  n737 = while {
    tunnel: w33 -> [_]
    tunnel: w17 -> [_]
    stop <- w992 stop-if-true
    # "New Adv Logics"
    n738 = local read "Main Tab"() -> (w972:T2)
    n739 = local read "Main Tab"() -> (w990:T2)
    n740 = local read "Sign In"() -> (w989:bool)
    n741 = case shown="\"Adv Scar\"" w972 {
      frame "HOME", Default {
        n742 = local read "LIVE FEED MIN TEMP"() -> (w1125:bool)
        n743 = local write "LIVE FEED MAX TEMP"(TRUE ("LIVE FEED MAX TEMP")) -> ()
        n744 = local read "CAMERA ROI MIN TEMP"() -> (w1123:bool)
        n745 = case shown="True" w1125 {
          selector: w1125 -> [_ w1132]
          frame False {
          }
          frame True {
            n746 = Not(x=w1132) -> (.not. x?=w1131:bool)
            n747 = local write "LIVE FEED MIN TEMP"(w1131) -> ()
            n748 = call "CAMERA LIVE FEED FGV.vi"("Enum - Menu"=CAMERA_LIVE_FEED_ENUM."CAMERA MINIMIZE") -> ()  [unwired: 9 in, 2 out]
          }
        }
        n749 = case shown="True" w1123 {
          selector: w1123 -> [_ w1129]
          frame False {
          }
          frame True {
            n750 = Not(x=w1129) -> (.not. x?=w1128:bool)
            n751 = local write "CAMERA ROI MIN TEMP"(w1128) -> ()
            n752 = call "IMAGE ANALYSIS.vi"("Enum"=POST_ANALYSIS_ENUM."MINIMIZE UI") -> ()  [unwired: 9 in, 2 out]
          }
        }
        n753 = local write "CAMERA ROI MAX TEMP"(TRUE ("CAMERA ROI MAX TEMP")) -> ()
      }
      frame "Test Setup" {
        n754 = local read "LIVE FEED MIN TEMP"() -> (w1135:bool)
        n755 = local read "CAMERA ROI MIN TEMP"() -> (w1133:bool)
        n756 = local write "LIVE FEED MAX TEMP"(TRUE ("LIVE FEED MAX TEMP")) -> ()
        n757 = case shown="True" w1135 {
          selector: w1135 -> [_ w1142]
          frame False {
          }
          frame True {
            n758 = Not(x=w1142) -> (.not. x?=w1141:bool)
            n759 = local write "LIVE FEED MIN TEMP"(w1141) -> ()
            n760 = call "CAMERA LIVE FEED FGV.vi"("Enum - Menu"=CAMERA_LIVE_FEED_ENUM."CAMERA MINIMIZE") -> ()  [unwired: 9 in, 2 out]
          }
        }
        n761 = case shown="True" w1133 {
          selector: w1133 -> [_ w1139]
          frame False {
          }
          frame True {
            n762 = Not(x=w1139) -> (.not. x?=w1138:bool)
            n763 = local write "CAMERA ROI MIN TEMP"(w1138) -> ()
            n764 = call "IMAGE ANALYSIS.vi"("Enum"=POST_ANALYSIS_ENUM."MINIMIZE UI") -> ()  [unwired: 9 in, 2 out]
          }
        }
        n765 = local write "CAMERA ROI MAX TEMP"(TRUE ("CAMERA ROI MAX TEMP")) -> ()
      }
      frame "Acquire" {
        n766 = local read "LIVE FEED MIN TEMP"() -> (w1145:bool)
        n767 = local write "LIVE FEED MAX TEMP"(TRUE ("LIVE FEED MAX TEMP")) -> ()
        n768 = local read "CAMERA ROI MIN TEMP"() -> (w1143:bool)
        n769 = case shown="True" w1145 {
          selector: w1145 -> [_ w1152]
          frame False {
          }
          frame True {
            n770 = Not(x=w1152) -> (.not. x?=w1151:bool)
            n771 = local write "LIVE FEED MIN TEMP"(w1151) -> ()
            n772 = call "CAMERA LIVE FEED FGV.vi"("Enum - Menu"=CAMERA_LIVE_FEED_ENUM."CAMERA MINIMIZE") -> ()  [unwired: 9 in, 2 out]
          }
        }
        n773 = case shown="True" w1143 {
          selector: w1143 -> [_ w1149]
          frame False {
          }
          frame True {
            n774 = Not(x=w1149) -> (.not. x?=w1148:bool)
            n775 = local write "CAMERA ROI MIN TEMP"(w1148) -> ()
            n776 = call "IMAGE ANALYSIS.vi"("Enum"=POST_ANALYSIS_ENUM."MINIMIZE UI") -> ()  [unwired: 9 in, 2 out]
          }
        }
        n777 = local write "CAMERA ROI MAX TEMP"(TRUE ("CAMERA ROI MAX TEMP")) -> ()
      }
      frame "Adv Scar" {
        n778 = local read "CAMERA ROI MIN TEMP"() -> (w1153:bool)
        n779 = case shown="True" "LIVE FEED MAX TEMP" {
          selector: "LIVE FEED MAX TEMP" -> [_ w1174]
          frame False {
          }
          frame True {
            n780 = Not(x=w1174) -> (.not. x?=w1173:bool)
            n781 = local write "LIVE FEED MAX TEMP"(w1173) -> ()
            n782 = call "CAMERA LIVE FEED FGV.vi"("Enum - Menu"=CAMERA_LIVE_FEED_ENUM."CAMERA RESTORE") -> ("error out"=w1164:errorcluster)  [unwired: 9 in, 1 out]
            n783 = Type Cast(type=30, x=0) -> (*(type *) &x=w1168:i32)
            n784 = Add(x=w1168, y=48) -> (x+y=w1169:i32)
            n785 = call "CAMERA LIVE FEED FGV.vi"("Enum - Menu"=CAMERA_LIVE_FEED_ENUM."CAMERA MODE SET", "error in (no error)"=w1164, "CAMERA MODE"=w1169) -> ("error out"=w1161:errorcluster)  [unwired: 7 in, 1 out]
            n786 = call "CAMERA LIVE FEED FGV.vi"("Enum - Menu"=CAMERA_LIVE_FEED_ENUM."CAMERA GRAY", "error in (no error)"=w1161) -> ("error out"=w1160:errorcluster)  [unwired: 8 in, 1 out]
            n787 = call "LIST FILE NAMES.vi"("error in (no error)"=w1160) -> ("error out"=w1170:errorcluster, "filenames"=w1171:string[])  [unwired: 9 in]
            n788 = property on="FILE 3" class="CmbBox"(error in=w1170, "Strings[]"=w1171) -> ()  [unwired: 1 in, 2 out]
          }
        }
        n789 = case shown="True" w1153 {
          selector: w1153 -> [_ w1159]
          frame False {
          }
          frame True {
            n790 = Not(x=w1159) -> (.not. x?=w1158:bool)
            n791 = local write "CAMERA ROI MIN TEMP"(w1158) -> ()
            n792 = call "IMAGE ANALYSIS.vi"("Enum"=POST_ANALYSIS_ENUM."MINIMIZE UI") -> ()  [unwired: 9 in, 2 out]
          }
        }
        n793 = local write "CAMERA ROI MAX TEMP"(TRUE ("CAMERA ROI MAX TEMP")) -> ()
        "LIVE FEED MIN TEMP" <- TRUE ("LIVE FEED MIN TEMP")
      }
      frame "Adv Scar Report" {
        n794 = local read "CAMERA ROI MAX TEMP"() -> (w1175:bool)
        n795 = local read "LIVE FEED MIN TEMP"() -> (w1177:bool)
